vi "Main_UDPsend.vi"() -> ()   [LabVIEW 2024]
doc: "This template is for the Queued Message Handler design pattern.\n\nThe Event Handling Loop generates messages based on user interface actions.\n\nThe Message Handling Loop processes messages generated by the Event Handling Loop, or by other messages. The messages are string values, so new messages can be added easily to the Message Cases case structure in the Message Handling Loop. Each message cluster can also provide an optional value for Message Data, which is a variant that can be converted to whatever message-specific data is required."
uses:
  support/Message Queue/Enqueue Message (Single).vi
  <vilib>/Utility/error.llb/Error Cluster From Error Code.vi
  <vilib>/ErrorRing/Error Ring.xnode
  support/Message Queue/Message Queue.lvlib
  support/User Event - Stop/User Event - Stop.lvlib
panel:
  in  "Stop":bool
  out "Received Data":dbl(graph)
  in  "Remote address":string="localhost"
  in  "Remote port":u16=61557
  out "Waveform Graph":dbl[](graph)
  out "Status":string
  in  "Acquire_Send":bool
  in  "Exit":bool
  # "UDP send lab 5"
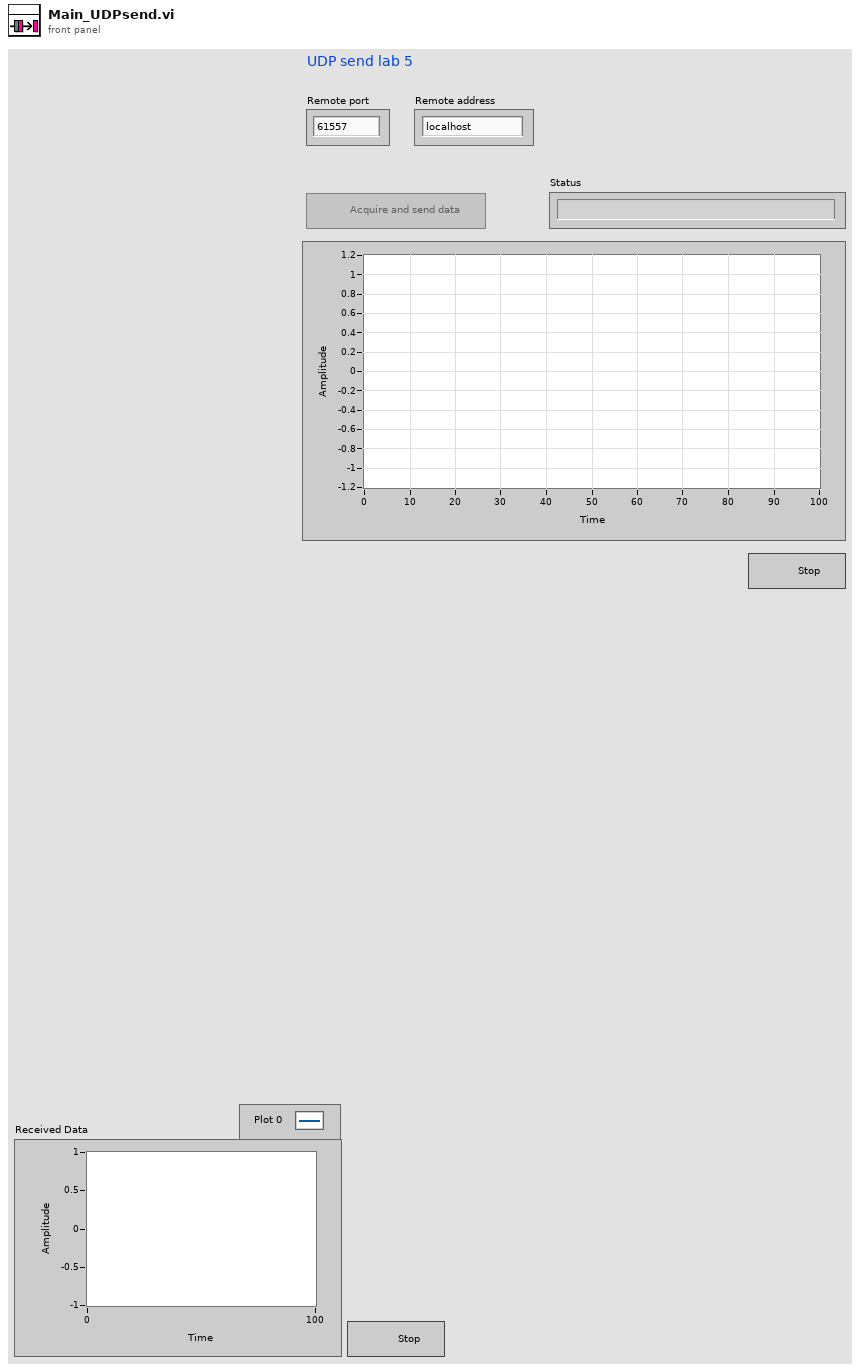
[diagram p1: front panel]
types:
  T1 = typedef "Message Queue.lvlib/All Message Queues.ctl" = cluster{"UI":refnum<queue>, "DAQ":refnum<queue>, "UDP":refnum<queue>}
  T2 = enum8{"Enabled", "Disabled", "Disabled and Grayed Out"}
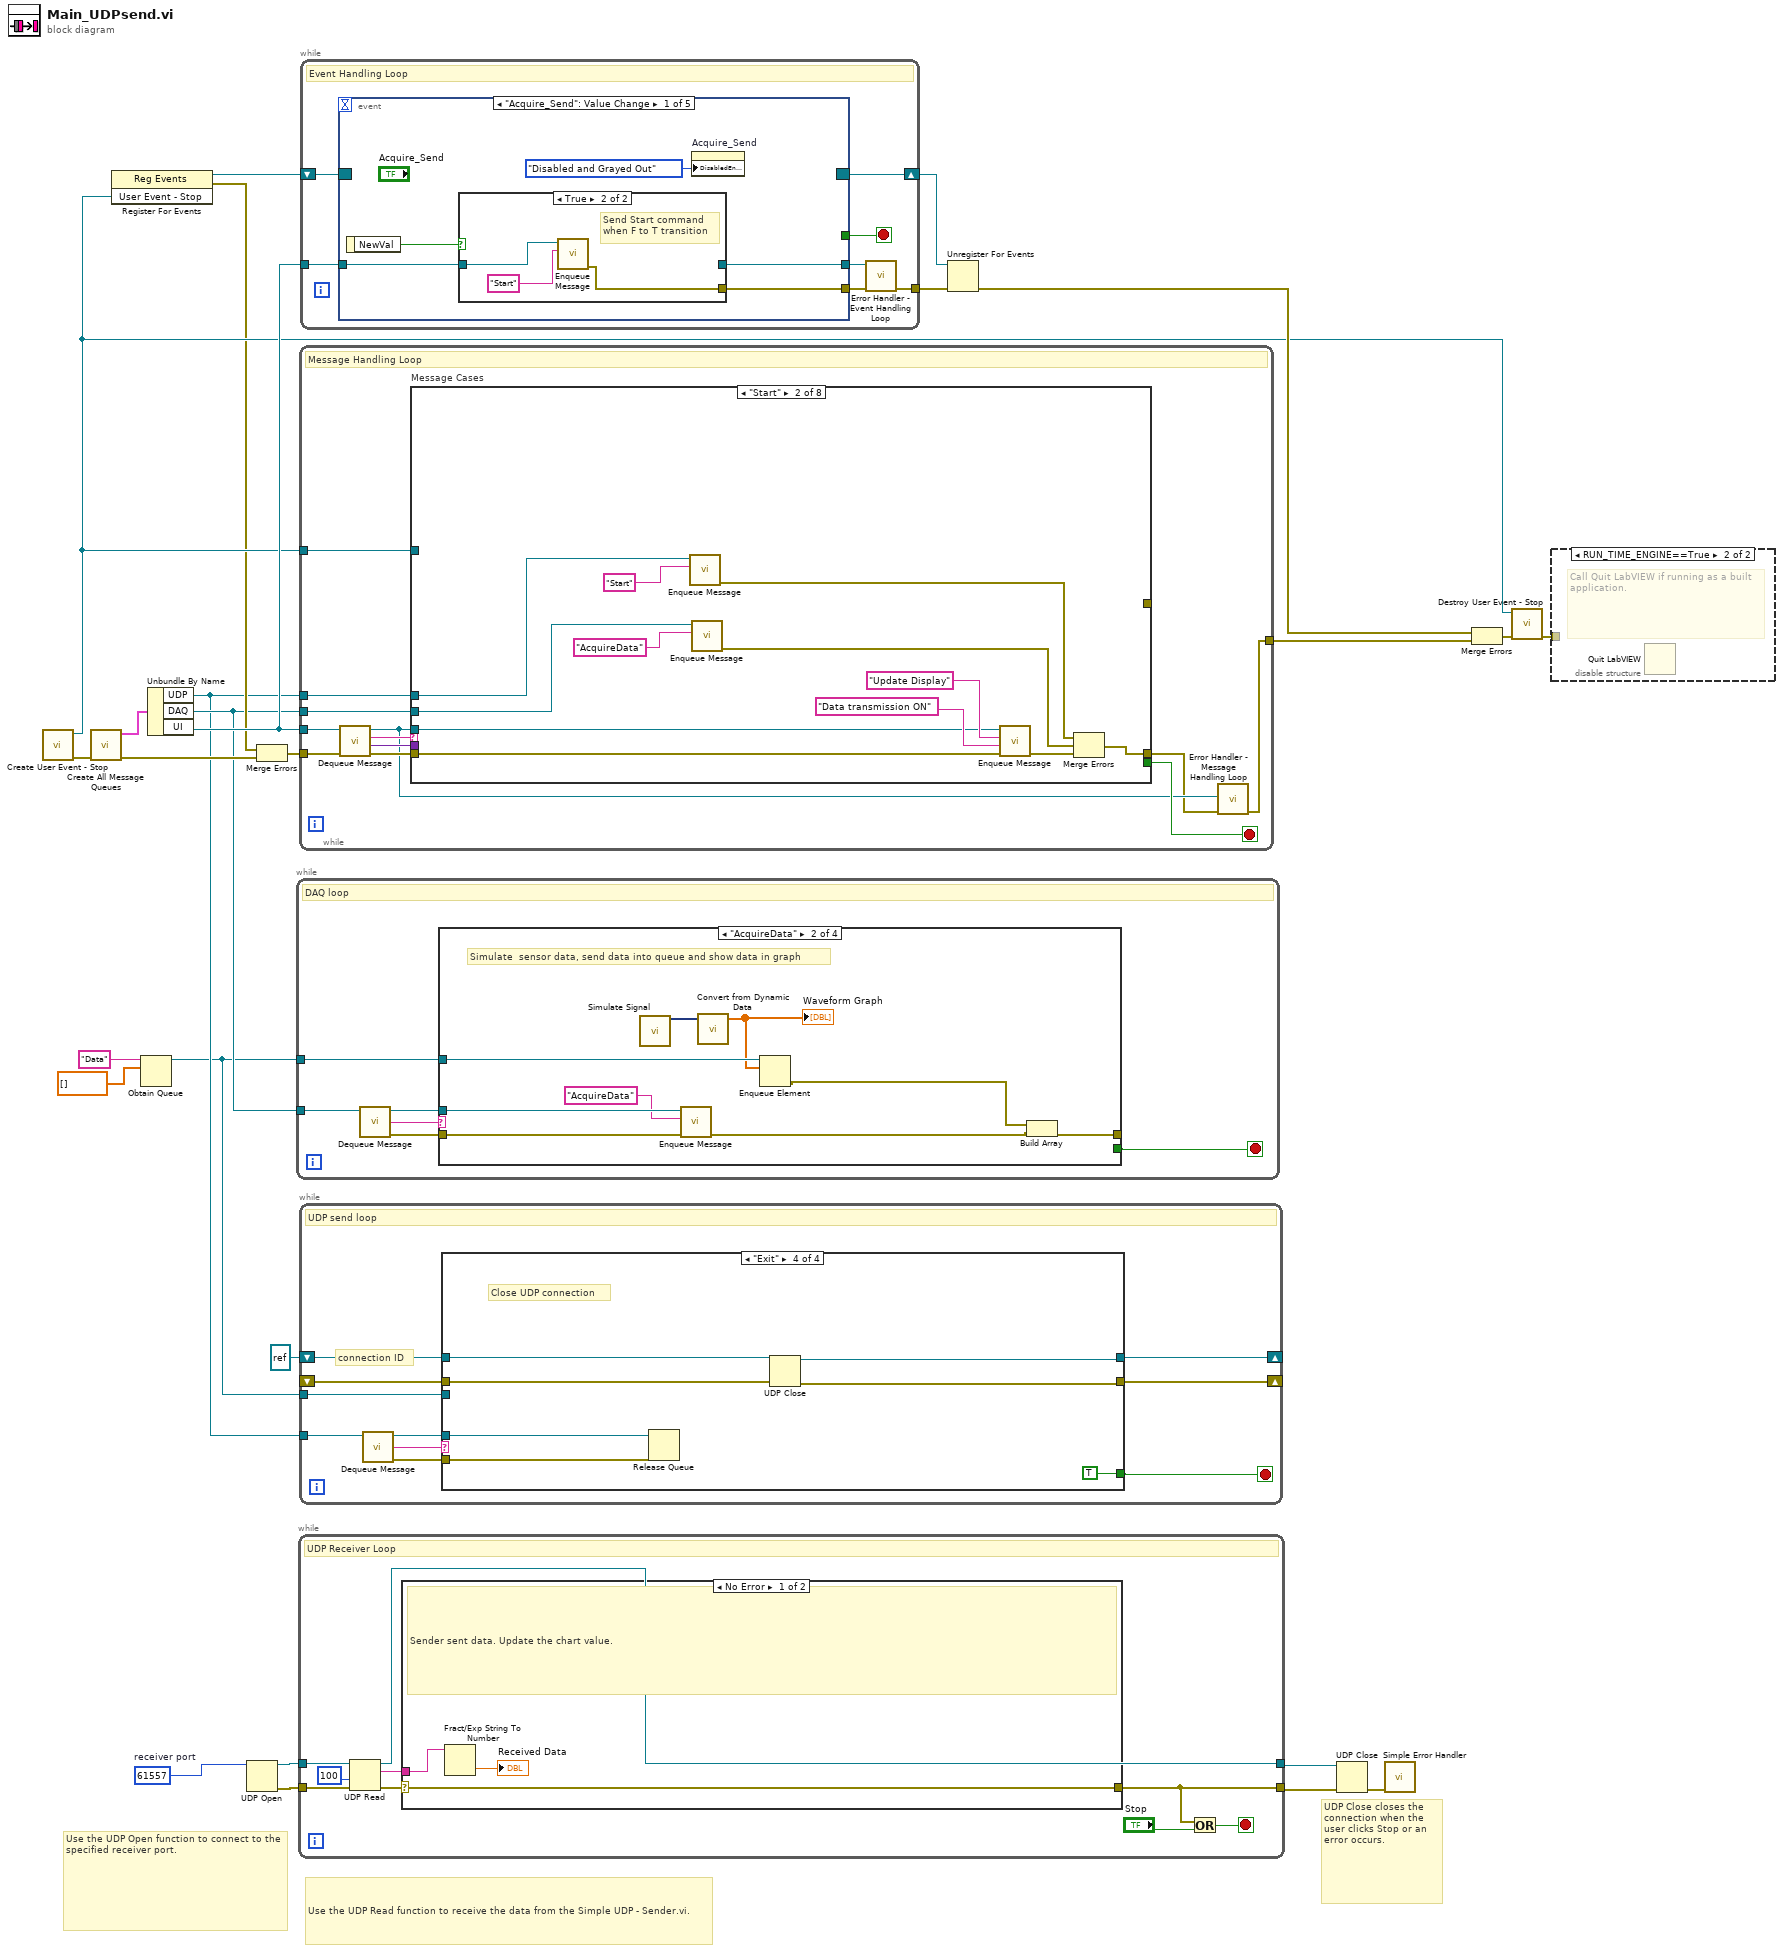
[diagram p0: block diagram]
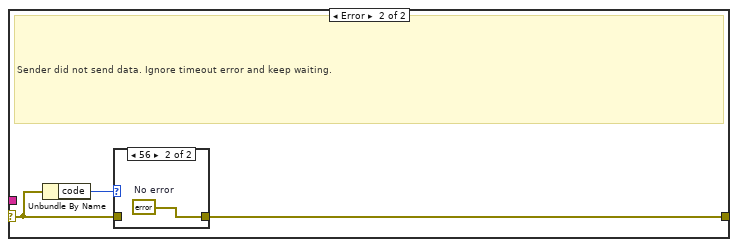
[diagram p2: hidden frame]
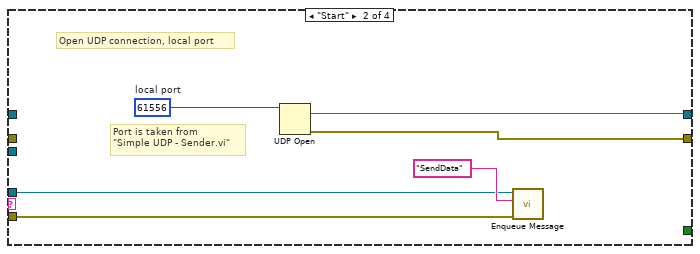
[diagram p5: hidden frame]
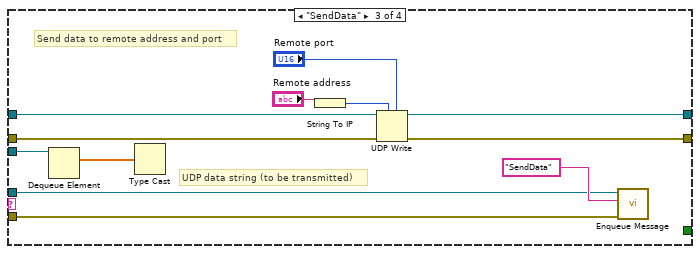
[diagram p6: hidden frame]
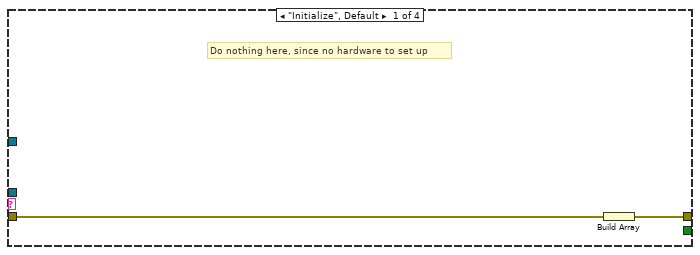
[diagram p7: hidden frame]
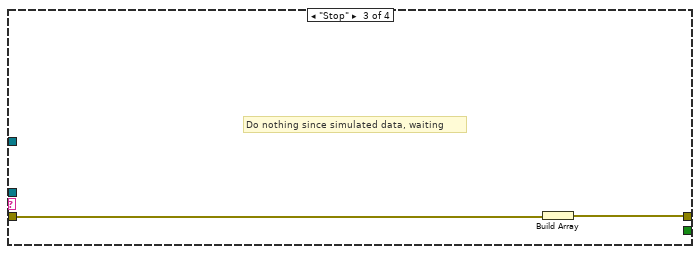
[diagram p8: hidden frame]
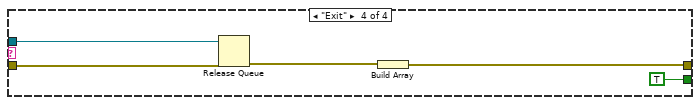
[diagram p9: hidden frame]
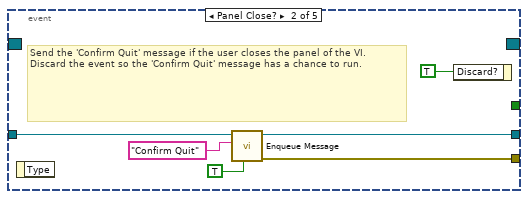
[diagram p12: hidden frame]
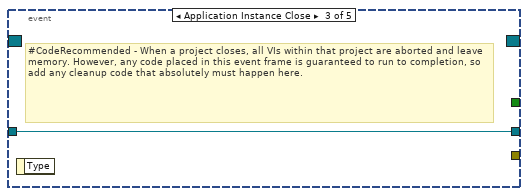
[diagram p13: hidden frame]
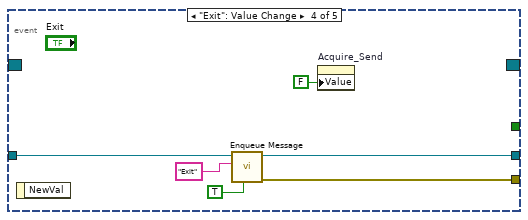
[diagram p14: hidden frame]
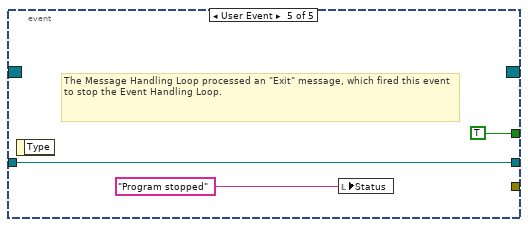
[diagram p15: hidden frame]
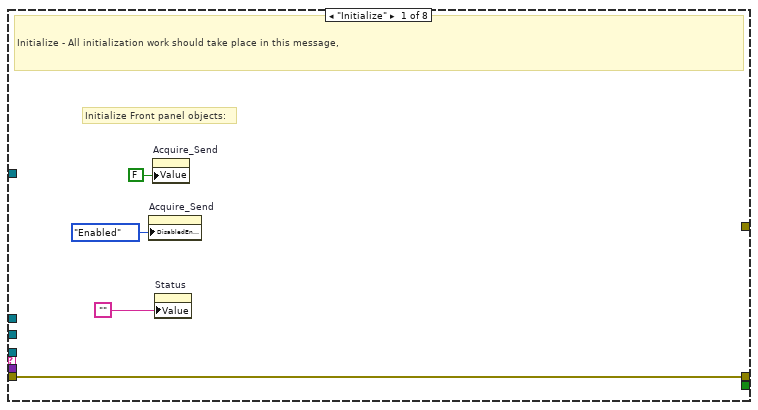
[diagram p16: hidden frame]
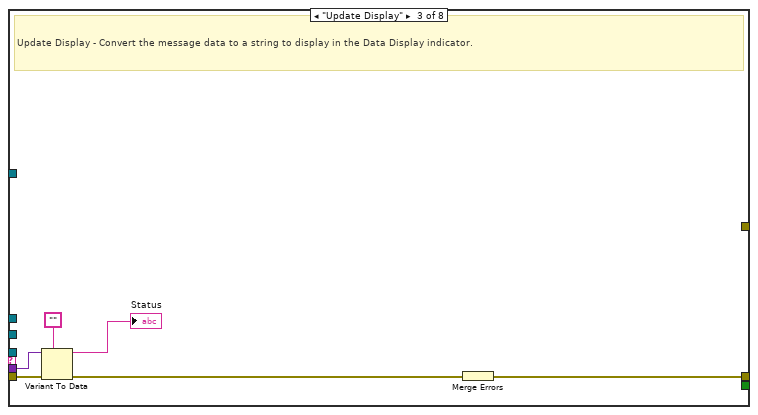
[diagram p17: hidden frame]
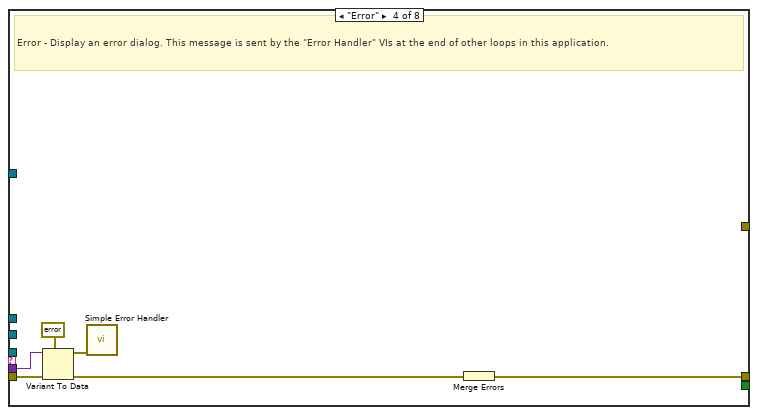
[diagram p18: hidden frame]
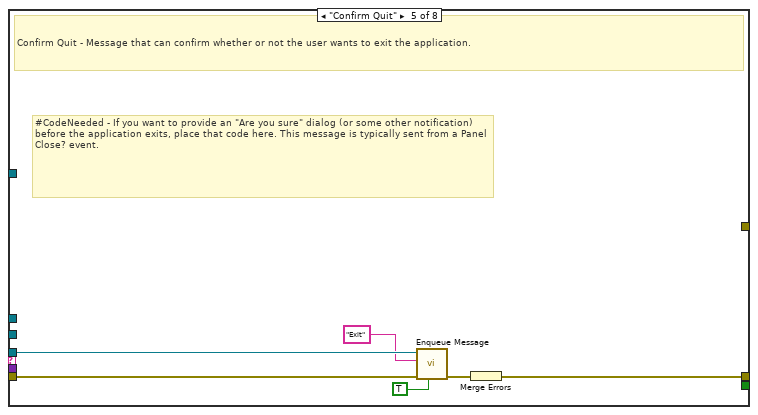
[diagram p19: hidden frame]
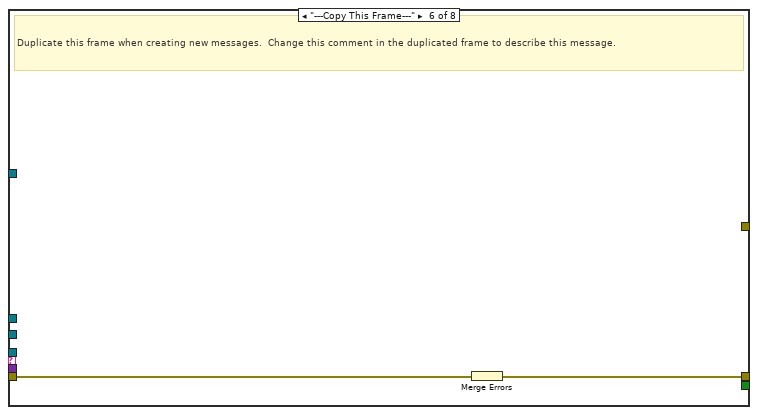
[diagram p20: hidden frame]
diagram:
  w1 = u16 61557  # receiver port
  # "UDP Close closes the connection when the user clicks Stop or an error occurs."
  # "Use the UDP Open function to connect to the specified receiver port."
  # "Use the UDP Read function to receive the data from the Simple UDP - Sender.vi."
  n1 = call "Create User Event - Stop.vi"() -> ("error out"=w22:errorcluster, "User Event - Stop"=w15:refnum<user-event>)  [unwired: 10 in]
  n2 = call "Create All Message Queues.vi"("error in (no error)"=w22) -> ("error out"=w26:errorcluster, "Message Queues out"=w25:T1)  [unwired: 9 in]
  n3 = register-events(w15) -> (reference out=w16:refnum<event-registration>, error out=w13:errorcluster)  [unwired: 2 in]
  n4 = Obtain Queue(name (unnamed)="Data", element data type=dbl[] [] ("Array")) -> (queue out=w7:refnum<queue>)  [unwired: 3 in, 2 out]
  n5 = Unbundle By Name(w25) -> ("UDP"=w9:refnum<queue>, "DAQ"=w12:refnum<queue>, "UI"=w23:refnum<queue>)
  n6 = UDP Open(11:w1) -> (port=w2:refnum<k16>, 0:w3:errorcluster)  [unwired: 4 in, 1 out]
  n7 = Merge Errors(w13, w26) -> (w14:errorcluster)
  n8 = while {
    tunnel: w12 -> [w31]
    tunnel: w7 -> [w28]
    stop <- w27 stop-if-true
    # "DAQ loop"
    n9 = call "Dequeue Message.vi"("Message Queue"=w31) -> ("error out"=w30:errorcluster, "Message"=w32:string, "dup Message Queue"=w29:refnum<queue>)  [unwired: 7 in, 1 out]
    n10 = case shown="\"AcquireData\"" w32 {
      tunnel: w30 -> [w34 w42 w44 w49]
      tunnel: [w33 w37 w45 w46] -> _
      tunnel: w29 -> [_ w41 _ w50]
      tunnel: w28 -> [_ w40 _ _]
      tunnel: [_ _ _ TRUE] -> w27
      frame "Initialize", Default {
        # "Do nothing here, since no hardware to set up"
        n11 = Build Array(w34) -> (w33:errorcluster[])
      }
      frame "AcquireData" {
        # "Simulate  sensor data, send data into queue and show data in graph"
        n12 = call "Simulate Signal"() -> ("Sine with Uniform Noise"=w43:dynamicdata)  [unwired: 14 in, 1 out]
        n13 = call-poly "Enqueue Message.vi"("error in (no error)"=w42, "Message"="AcquireData", "Message Queue"=w41) -> ("error out"=w38:errorcluster)  [unwired: 7 in, 1 out]
        n14 = call "Convert from Dynamic Data"("Dynamic Data Type"=w43) -> ("Array"=w39:dbl[])  [unwired: 3 in]
        "Waveform Graph" <- w39
        n15 = Enqueue Element(queue=w40, element=w39) -> (error out=w36:errorcluster)  [unwired: 2 in, 2 out]
        n16 = Build Array(w36, w38) -> (w37:errorcluster[])
      }
      frame "Stop" {
        # "Do nothing since simulated data, waiting"
        n17 = Build Array(w44) -> (w45:errorcluster[])
      }
      frame "Exit" {
        n18 = Release Queue(queue=w50, error in (no error)=w49) -> (error out=w47:errorcluster)  [unwired: 1 in, 2 out]
        n19 = Build Array(w47) -> (w46:errorcluster[])
      }
    }
  }
  n20 = while {
    tunnel: w2 -> [w59]
    tunnel: [w51] -> w6
    tunnel: w3 -> [w56]
    tunnel: [w52] -> w4
    stop <- w57 stop-if-true
    # "UDP Receiver Loop"
    n21 = UDP Read(connection ID=w59, timeout ms (25000)=100, 8:w56) -> (data out=w54:string, error out=w53:errorcluster, 3:w51:refnum<k16>)  [unwired: 3 out]
    n22 = case shown="No Error" w53 {
      selector: w53 -> [w60 w64]
      tunnel: w54 -> [w62 _]
      tunnel: [w60 w63] -> w52
      frame No Error {
        # "Sender sent data. Update the chart value."
        n23 = Fract/Exp String To Number(string=w62) -> (number=→"Received Data":dbl)  [unwired: 3 in, 1 out]
      }
      frame Error {
        # "Sender did not send data. Ignore timeout error and keep waiting."
        n24 = Unbundle By Name(w64) -> ("code"=w65:i32)
        n25 = case shown="56" w65 {
          tunnel: w64 -> [w66 _]
          tunnel: [w66 w67] -> w63
          frame Default {
          }
          frame 56 {
            w67 = errorcluster {"status"=FALSE, "code"=0, "source"=""}  # No error
          }
        }
      }
    }
    n26 = Or(x=w52, y="Stop") -> (x .or. y?=w57:bool)
  }
  n27 = while {
    tunnel: w23 -> [w73]
    tunnel: w15 -> [w78]
    tunnel: w14 -> [w77]
    tunnel: [w71] -> w24
    tunnel: w12 -> [w69]
    tunnel: w9 -> [w68]
    stop <- w79 stop-if-true
    # "Message Handling Loop"
    n28 = call "Dequeue Message.vi"("error in (no error)"=w77, "Message Queue"=w73) -> ("error out"=w76:errorcluster, "Message Data"=w74:variant, "Message"=w75:string, "dup Message Queue"=w72:refnum<queue>)  [unwired: 6 in]
    n29 = case "Message Cases" shown="\"Start\"" w75 {
      selector: w75 -> [_ _ _ _ _ _ _ w132]
      tunnel: w72 -> [_ w90 _ _ w110 _ w131 _]
      tunnel: w76 -> [w83 w89 w100 w107 w113 w115 w125 _]
      tunnel: [w83 w95 w101 w102 w112 w114 w128 w133] -> w70
      tunnel: [_ _ _ _ _ _ TRUE _] -> w79
      tunnel: w74 -> [_ _ w99 w106 _ _ w122 _]
      tunnel: w78 -> [_ _ _ _ _ _ w127 _]
      tunnel: w69 -> [_ w88 _ _ _ _ w117 _]
      tunnel: w68 -> [_ w86 _ _ _ _ w120 _]
      tunnel: [_ _ _ _ _ _ w116 _] -> _
      frame "Initialize" {
        # "Initialize Front panel objects:"
        # "Initialize - All initialization work should take place in this message,"
        n30 = property on="Acquire_Send" class="Bool (strict)"("DisabledEnum"=T2."Enabled" ("Disabled")) -> ()  [unwired: 2 in, 2 out]
        n31 = property on="Acquire_Send" class="Bool (strict)"("Value"=FALSE ("Acquire_Send")) -> ()  [unwired: 2 in, 2 out]
        n32 = property on="Status" class="Str"("Value"="") -> ()  [unwired: 2 in, 2 out]
      }
      frame "Start" {
        n33 = call-poly "Enqueue Message.vi"("Message"="Start", "Message Queue"=w86) -> ("error out"=w84:errorcluster)  [unwired: 8 in, 1 out]
        n34 = call-poly "Enqueue Message.vi"("Message"="AcquireData", "Message Queue"=w88) -> ("error out"=w85:errorcluster)  [unwired: 8 in, 1 out]
        n35 = call-poly "Enqueue Message.vi"("error in (no error)"=w89, "Message Data"="Data transmission ON" ("\"Do Something\" button pressed"), "Message"="Update Display", "Message Queue"=w90) -> ("error out"=w94:errorcluster)  [unwired: 6 in, 1 out]
        n36 = Merge Errors "Merge Errors"(w84, w85, w94) -> (w95:errorcluster)
      }
      frame "Update Display" {
        # "Update Display - Convert the message data to a string to display in the Data Display indicator."
        n37 = Variant To Data(error in=w100, type="", Variant=w99) -> (data=→"Status":string, error out=w97:errorcluster)
        n38 = Merge Errors(w97) -> (w101:errorcluster)
      }
      frame "Error" {
        # "Error - Display an error dialog. This message is sent by the \"Error Handler\" VIs at the end of other loops in this application."
        n39 = Variant To Data(error in=w107, type=errorcluster {"status"=FALSE, "code"=0, "source"=""} ("error constant"), Variant=w106) -> (data=w104:errorcluster, error out=w103:errorcluster)
        n40 = call <vilib>:"Simple Error Handler.vi"("error in (no error)"=w104) -> ()  [unwired: 4 in, 5 out]
        n41 = Merge Errors(w103) -> (w102:errorcluster)
      }
      frame "Confirm Quit" {
        # "#CodeNeeded - If you want to provide an \"Are you sure\" dialog (or some other notification) before the application exits, place that code here. This message is typically sent from a Panel Close? event."
        # "Confirm Quit - Message that can confirm whether or not the user wants to exit the application."
        n42 = call-poly "Enqueue Message.vi"("Priority Message? (F)"=TRUE, "error in (no error)"=w113, "Message"="Exit", "Message Queue"=w110) -> ("error out"=w111:errorcluster)  [unwired: 6 in, 1 out]
        n43 = Merge Errors(w111) -> (w112:errorcluster)
      }
      frame "---Copy This Frame---" {
        # "Duplicate this frame when creating new messages.  Change this comment in the duplicated frame to describe this message."
        n44 = Merge Errors(w115) -> (w114:errorcluster)
      }
      frame "Exit" {
        w121 = "Exit" ("Message")
        # "Stop the VI"
        # "Release the message queue reference"
        # "Exit - Exit the application."
        n45 = Flush Queue(queue=w117) -> (queue out=w118:refnum<queue>)  [unwired: 1 in, 2 out]
        n46 = Flush Queue(queue=w120) -> (queue out=w119:refnum<queue>)  [unwired: 1 in, 2 out]
        n47 = call-poly "Enqueue Message.vi"("Message"=w121, "Message Queue"=w119) -> ("error out"=w116:errorcluster)  [unwired: 8 in, 1 out]
        n48 = call-poly "Enqueue Message.vi"("Message"=w121, "Message Queue"=w118) -> ()  [unwired: 8 in, 2 out]
        n49 = Variant To Data(type=errorcluster {"status"=FALSE, "code"=0, "source"=""} ("error constant"), Variant=w122) -> (data=w123:errorcluster)  [unwired: 1 in, 1 out]
        n50 = call <vilib>:"Simple Error Handler.vi"("error in (no error)"=w123) -> ()  [unwired: 4 in, 5 out]
        n51 = Release Queue(queue=w131, error in (no error)=w125) -> (error out=w129:errorcluster)  [unwired: 1 in, 2 out]
        n52 = call "Fire User Event - Stop.vi"("User Event - Stop"=w127) -> ("error out"=w126:errorcluster)  [unwired: 10 in]
        n53 = Merge Errors(w126, w129) -> (w128:errorcluster)
      }
      frame Default {
        # "'Default' case only runs if there is a message that isn't defined in any of the other cases.  Output a programming error."
        n54 = xnode "Error Ring"("parameter 0"=w132) -> ("error out"=w133:errorcluster)
      }
    }
    n55 = call "Error Handler - Message Handling Loop.vi"("error in (no error)"=w70, "Message Queue"=w72) -> ("dup error in"=w71:errorcluster)  [unwired: 8 in, 1 out]
  }
  n56 = while {
    tunnel: w9 -> [w149]
    shift-right: [w145] -> _
    shift-left: refnum<k16> refnum ("port") -> [w144]
    tunnel: w7 -> [w143]
    shift-right: [w142] -> _
    shift-left: _ -> [w141]
    stop <- w146 stop-if-true
    # "connection ID"
    # "UDP send loop"
    n57 = call "Dequeue Message.vi"("Message Queue"=w149) -> ("error out"=w148:errorcluster, "Message"=w150:string, "dup Message Queue"=w147:refnum<queue>)  [unwired: 7 in, 1 out]
    n58 = case shown="\"Exit\"" w150 {
      tunnel: w148 -> [w151 w157 w169 w176]
      tunnel: w147 -> [_ w156 w168 w177]
      tunnel: [_ _ _ TRUE] -> w146
      tunnel: [w152 w154 w159 w173] -> w145
      tunnel: w144 -> [w152 _ w162 w174]
      tunnel: w143 -> [_ _ w166 _]
      tunnel: [w151 w153 w160 w171] -> w142
      tunnel: w141 -> [_ _ w161 w172]
      frame "Initialize", Default {
        # "Nothing done here"
      }
      frame "Start" {
        w155 = 61556  # local port
        # "Port is taken from \n\"Simple UDP - Sender.vi\""
        # "Open UDP connection, local port"
        n59 = UDP Open(11:w155) -> (port=w154:refnum<k16>, 0:w153:errorcluster)  [unwired: 4 in, 1 out]
        n60 = call-poly "Enqueue Message.vi"("error in (no error)"=w157, "Message"="SendData", "Message Queue"=w156) -> ()  [unwired: 7 in, 2 out]
      }
      frame "SendData" {
        # "UDP data string (to be transmitted)"
        # "Send data to remote address and port"
        n61 = Dequeue Element(queue=w166) -> (element=w165:dbl[])  [unwired: 2 in, 3 out]
        n62 = Type Cast(x=w165) -> ()  [unwired: 1 in, 1 out]
        n63 = String To IP(1:"Remote address") -> (0:w164:u32)
        n64 = UDP Write(address=w164, port or service name="Remote port", connection ID=w162, 8:w161) -> (error out=w160:errorcluster, 3:w159:refnum<k16>)  [unwired: 2 in]
        n65 = call-poly "Enqueue Message.vi"("error in (no error)"=w169, "Message"="SendData", "Message Queue"=w168) -> ()  [unwired: 7 in, 2 out]
      }
      frame "Exit" {
        # "Close UDP connection"
        n66 = Release Queue(queue=w177, error in (no error)=w176) -> ()  [unwired: 1 in, 3 out]
        n67 = UDP Close(connection ID=w174, 8:w172) -> (connection ID out=w173:refnum<k16>, error out=w171:errorcluster)
      }
    }
  }
  n68 = while {
    tunnel: w23 -> [w184]
    shift-right: [w182] -> w19
    shift-left: w16 -> [w183]
    tunnel: [w178] -> w17
    stop <- w180 stop-if-true
    # "Event Handling Loop"
    n69 = event shown="[0] \"Acquire_Send\": Value Change" {
      selector: w183 -> [_ _ _ _ _]
      dyn-events: [_ _ _ _ _] -> w182
      timeout: _ -> [_ _ _ _ _]
      tunnel: [_ _ _ _ TRUE ("Discard?")] -> w180
      tunnel: w184 -> [w189 w198 w200 w206 w209]
      tunnel: [w187 w197 _ w205 _] -> w181
      tunnel: [w188 w196 w200 w204 w209] -> w179
      event "Acquire_Send": Value Change {
        n70 = event-data() -> ("NewVal"=w185:bool)  [unwired: 1 in]
        n71 = case shown="True" w185 {
          tunnel: w189 -> [w190 w192]
          tunnel: [w190 _] -> w188
          tunnel: [_ w191] -> w187
          frame False {
          }
          frame True {
            # "Send Start command \nwhen F to T transition"
            n72 = call-poly "Enqueue Message.vi"("Message"="Start", "Message Queue"=w192) -> ("error out"=w191:errorcluster)  [unwired: 8 in, 1 out]
          }
        }
        n73 = property on="Acquire_Send" class="Bool (strict)"("DisabledEnum"=T2."Disabled and Grayed Out" ("Disabled")) -> ()  [unwired: 2 in, 2 out]
      }
      event Panel Close? {
        # "Send the 'Confirm Quit' message if the user closes the panel of the VI. Discard the event so the 'Confirm Quit' message has a chance to run."
        n74 = event-data() -> ()  [unwired: 1 in, 1 out]
        n75 = call-poly "Enqueue Message.vi"("Priority Message? (F)"=TRUE, "Message"="Confirm Quit", "Message Queue"=w198) -> ("error out"=w197:errorcluster, "dup Message Queue"=w196:refnum<queue>)  [unwired: 7 in]
        n76 = event-data("Discard?"=TRUE) -> ()  [unwired: 1 in, 1 out]
      }
      event Application Instance Close {
        # "#CodeRecommended - When a project closes, all VIs within that project are aborted and leave memory. However, any code placed in this event frame is guaranteed to run to completion, so add any cleanup code that absolutely must happen here."
        n77 = event-data() -> ()  [unwired: 1 in, 1 out]
      }
      event "Exit": Value Change {
        n78 = event-data() -> ()  [unwired: 1 in, 1 out]
        n79 = call-poly "Enqueue Message.vi"("Priority Message? (F)"=TRUE, "Message"="Exit", "Message Queue"=w206) -> ("error out"=w205:errorcluster, "dup Message Queue"=w204:refnum<queue>)  [unwired: 7 in]
        n80 = property on="Acquire_Send" class="Bool (strict)"("Value"=FALSE ("Acquire_Send")) -> ()  [unwired: 2 in, 2 out]
      }
      event User Event {
        # "The Message Handling Loop processed an \"Exit\" message, which fired this event to stop the Event Handling Loop."
        n81 = event-data() -> ()  [unwired: 1 in, 1 out]
        n82 = local write "Status"("Program stopped" ("VI Stopped")) -> ()
      }
    }
    n83 = call "Error Handler - Event Handling Loop.vi"("error in (no error)"=w181, "Message Queue"=w179) -> ("dup error in"=w178:errorcluster)  [unwired: 8 in, 1 out]
  }
  n84 = Unregister For Events(event registration refnum=w19, error in=w17) -> (error out=w20:errorcluster)
  n85 = UDP Close(connection ID=w6, 8:w4) -> (error out=w5:errorcluster)  [unwired: 1 out]
  n86 = call <vilib>:"Simple Error Handler.vi"("error in (no error)"=w5) -> ()  [unwired: 1 in, 8 out]
  n87 = Merge Errors(w20, w24) -> (w21:errorcluster)
  n88 = call "Destroy User Event - Stop.vi"("error in (no error)"=w21, "User Event - Stop"=w15) -> ("error out"=w18:errorcluster)  [unwired: 9 in]
  n89 = disable-structure shown="RUN_TIME_ENGINE==True" {
    disable-tunnel: w18 -> [_ _]
    frame condition #0 (active) {
    }
    frame condition #1 {
      # "Call Quit LabVIEW if running as a built application."
      n90 = Quit LabVIEW() -> ()  [unwired: 1 in]
    }
  }
